vi "DPT File AI Stream Save.vi"(9 "Stream Data Input":string[][](array[string]), 10 "Input Data Array":dbl[][](array[numeric]), 11 "Enable":bool) -> (1 "Voltage Stream Header Out":string[][](array[string]), 2 "Time":string, 3 "Stream Data":string[][](array[string]))   [LabVIEW 2014]
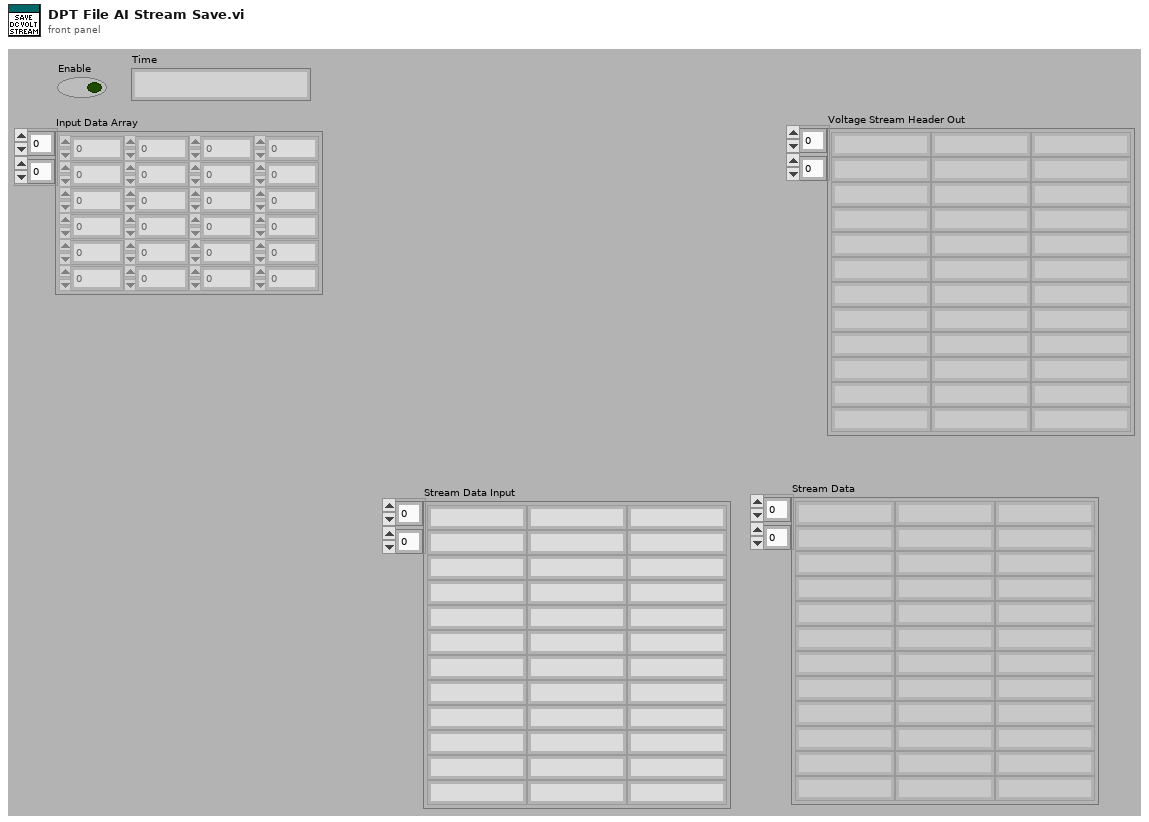
[diagram p1: front panel]
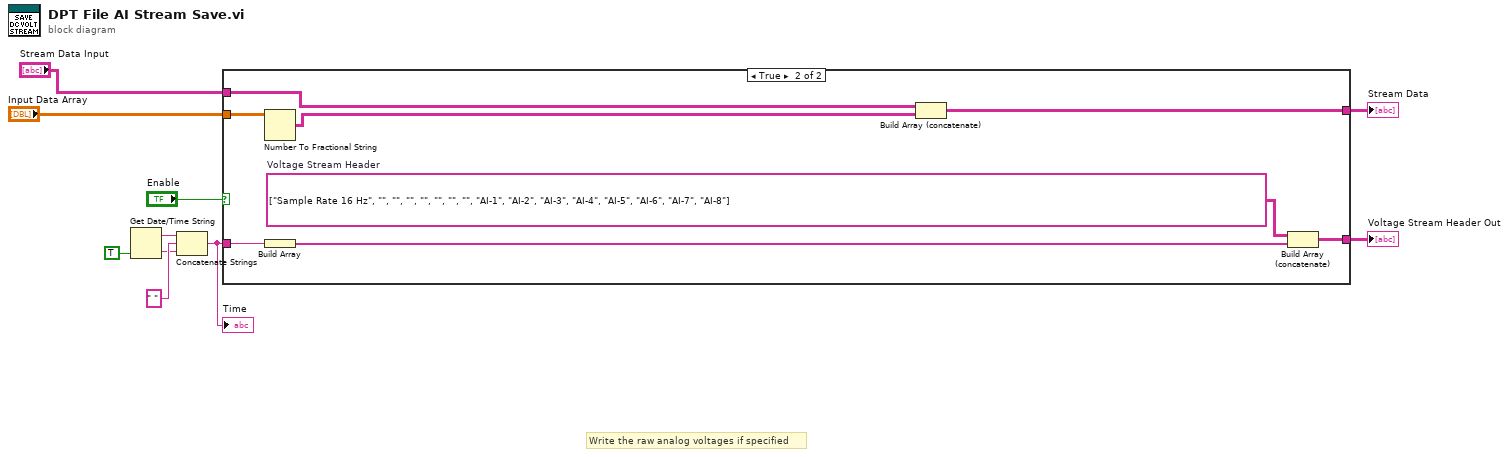
[diagram p0: block diagram]
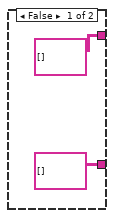
[diagram p2: hidden frame]
diagram:
  # "Write the raw analog voltages if specified"
  n1 = Get Date/Time String(want seconds? (F)=TRUE) -> (date string=w6:string, time string=w5:string)  [unwired: 2 in]
  n2 = Concatenate Strings(w6, " " ("string"), w5) -> (w4:string)
  "Time" <- w4
  n3 = case shown="True" "Enable" {
    tunnel: "Input Data Array" -> [_ w20]
    tunnel: w4 -> [_ w18]
    tunnel: [string[][] [] w13] -> w2
    tunnel: [string[][] [] w16] -> w3
    tunnel: "Stream Data Input" -> [_ w15]
    frame False {
    }
    frame True {
      w19 = string[][] [["Sample Rate 16 Hz", "", "", "", "", "", "", ""], ["AI-1", "AI-2", "AI-3", "AI-4", "AI-5", "AI-6", "AI-7", "AI-8"]]  # Voltage Stream Header
      n4 = Number To Fractional String(number=w20) -> (F-format string=w14:string[][])  [unwired: 3 in]
      n5 = Build Array(w18) -> (w17:string[])
      n6 = Build Array (concatenate)(w15, w14) -> (w13:string[][])
      n7 = Build Array (concatenate)(w19, w17) -> (w16:string[][])
    }
  }
  "Voltage Stream Header Out" <- w3
  "Stream Data" <- w2
